vi "Query.vi"(8 "error in (no error)":errorcluster, 9 "current time":timestamp, 10 "gRPCid":T4, 11 "HVC9 In":T1) -> (0 "error out":errorcluster, 3 "HVC9 Out":T1)   [LabVIEW 2019, in "HVC9 User.lvlib"]
uses:
  HVC9 User.lvlib
  Servers/HVC9/gRPC lvSupport/Server API/typeDefs/grpcId.ctl
  Types/HVC9.ctl
  Types/HVC9 gRPC IDs.ctl
  Types/HVC9 Data.ctl
  Servers/HVC9/HVC9 Class/RPC Messages/measurementservice_QueryResponse/measurementservice_QueryResponse_Data.ctl
  Servers/HVC9/HVC9 Class/HVC9.lvclass
  Servers/HVC9/gRPC lvSupport/gprc-lvsupport.lvlib
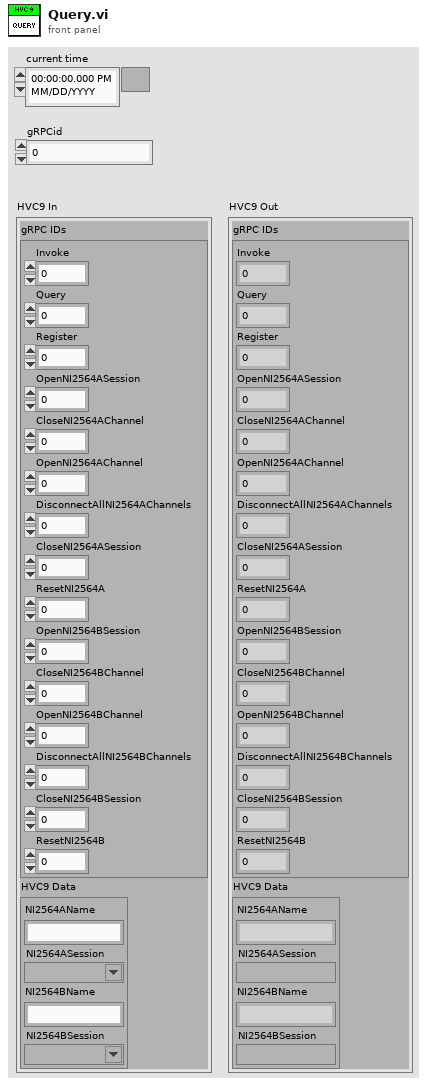
[diagram p1: front panel]
types:
  T1 = typedef "HVC9 User.lvlib/HVC9.ctl" = cluster{"gRPC IDs":T2, "HVC9 Data":T3}
  T2 = typedef "HVC9 User.lvlib/HVC9 gRPC IDs.ctl" = cluster{"Invoke ":u32, "Query":u32, "Register":u32, "OpenNI2564ASession":u32, "CloseNI2564AChannel ":u32, "OpenNI2564AChannel":u32, "DisconnectAllNI2564AChannels":u32, "CloseNI2564ASession":u32, "ResetNI2564A":u32, "OpenNI2564BSession":u32, "CloseNI2564BChannel ":u32, "OpenNI2564BChannel":u32, "DisconnectAllNI2564BChannels":u32, "CloseNI2564BSession":u32, "ResetNI2564B":u32}
  T3 = typedef "HVC9 User.lvlib/HVC9 Data.ctl" = cluster{"NI2564AName":string, "NI2564ASession":refnum<k15>, "NI2564BName":string, "NI2564BSession":refnum<k15>}
  T4 = typedef "HVC9.lvlib/gprc-lvsupport.lvlib/grpcId.ctl" = u64
  T5 = typedef "HVC9.lvlib/HVC9.lvclass/measurementservice_QueryResponse_Data.ctl" = cluster{"message":string, "status":i32}
  T6 = typedef "HVC9.lvlib/HVC9.lvclass/measurementservice_QueryRequest_Data.ctl" = cluster{"query":string}
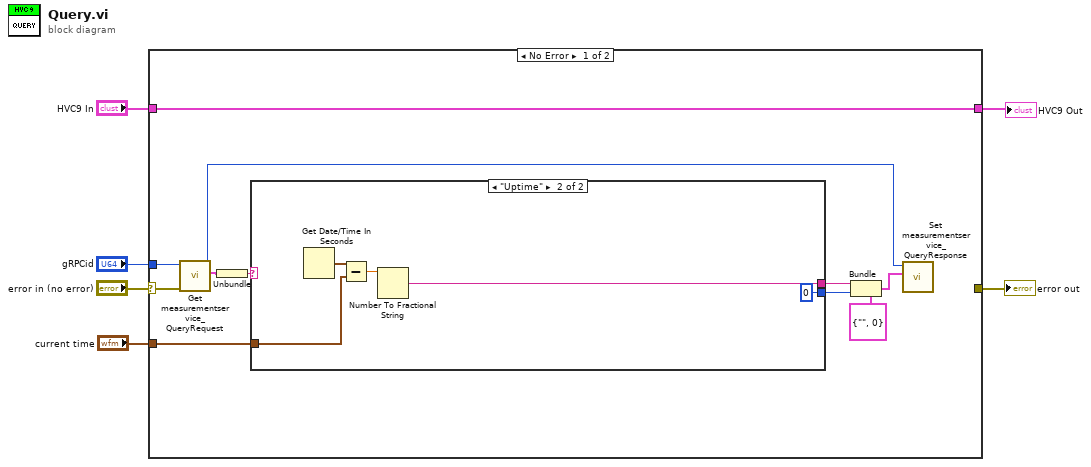
[diagram p0: block diagram]
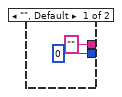
[diagram p2: hidden frame]
diagram:
  n1 = case shown="No Error" "error in (no error)" {
    selector: "error in (no error)" -> [w16 w25]
    tunnel: [w7 w26] -> w2
    tunnel: "HVC9 In" -> [w7 w26]
    tunnel: "gRPCid" -> [w17 _]
    tunnel: [_ w25] -> w5
    tunnel: "current time" -> [w13 _]
    frame No Error {
      n2 = call "Get measurementservice_QueryRequest.vi"("error in (no error)"=w16, "gRPCid"=w17) -> ("Message Data"=w15:T6, "gRPCid out"=w12:T4)  [unwired: 7 in, 1 out]
      n3 = Unbundle(w15) -> ("query"=w14:string)
      n4 = case shown="\"Uptime\"" w14 {
        tunnel: w13 -> [_ w23]
        tunnel: ["" w21] -> w9
        tunnel: [0 ("status") 0 ("status")] -> w8
        frame "", Default {
        }
        frame "Uptime" {
          n5 = Get Date/Time In Seconds() -> (seconds since 1Jan1904=w24:timestamp)
          n6 = Subtract(x=w24, y=w23) -> (x-y=w22:dbl)
          n7 = Number To Fractional String(number=w22) -> (F-format string=w21:string)  [unwired: 3 in]
        }
      }
      n8 = Bundle(cluster=T5 {"message"="", "status"=0} ("measurementservice_QueryResponse_Data"), "message"=w9, "status"=w8) -> (w11:T5)
      n9 = call "Set measurementservice_QueryResponse.vi"("Message Data"=w11, "gRPCid"=w12) -> ()  [unwired: 9 in, 1 out]
    }
    frame Error {
    }
  }
  "error out" <- w5
  "HVC9 Out" <- w2
